vi "Keyence.Main.vi"(11 "idx":i32) -> ()   [LabVIEW 2016]
uses:
  Keyence.Data.ctl
  Keyence.Data.Status.ctl
  Keyence.Data.Status.State.ctl
  Keyence.Data.Sets.ctl
  LowLevel/Keyence.CodeDetails.ctl
  Keyence.Action.ctl
  tools/CitTemplate/citTemplate.errData.ctl
  tools/EventLog/EventLog.EventSource.ctl
  Global/ApplicationGlobal.vi
  LowLevel/Keyence.Global.vi
panel:
  out "Action":T1=enum."--- Keyence ---"
  out "Data":T2={"Status"={"State"=enum."Init", "Ref"=refnum, "Bank"=0, "Version"="", "Model"="", "EndTS"=timestamp(0 s since 1904-01-01), "ImgPath"=path "", "Tuned"=FALSE}, "Sets"={"IP"="192.168.2.1", "Timeout_ms"=5000, "Retries"=0, "ReconnectPeriod_s"=0, "ResetPeriod_s"=0, "ReadImg"=FALSE}, "Code"={"text"="", "status"=FALSE, "corners"=[], "level"=0, "class"="", "path"=path ""}}
  out "_loop":i32(ring)=4
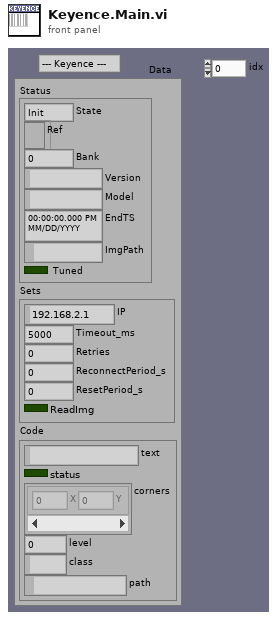
[diagram p1: front panel]
types:
  T1 = typedef "Keyence.Action.ctl" = enum32{"idle", "constructor", "destructor", "--- Keyence ---", "Init", "Scan", "Tune"}
  T2 = typedef "Keyence.Data.ctl" = cluster{"Status":T3, "Sets":T5, "Code":T6}
  T3 = typedef "Keyence.Data.Status.ctl" = cluster{"State":T4, "Ref":refnum<k5>, "Bank":u8, "Version":string, "Model":string, "EndTS":timestamp, "ImgPath":path, "Tuned":bool}
  T4 = typedef "Keyence.Data.Status.State.ctl" = enum16{"First", "Init", "Reset", "Idle", "Scan", "Tune"}
  T5 = typedef "Keyence.Data.Sets.ctl" = cluster{"IP":string, "Timeout_ms":i32, "Retries":i32, "ReconnectPeriod_s":i32, "ResetPeriod_s":i32, "ReadImg":bool}
  T6 = typedef "Keyence.CodeDetails.ctl" = cluster{"text":string, "status":bool, "corners":cluster{"X":i32, "Y":i32}[], "level":u8, "class":string, "path":path}
  T7 = typedef "EventLog.EventSource.ctl" = enum16{"All", "Gui", "Ref", "File", "Arch", "Seq", "CPX", "DB", "Laser", "Scan.P", "Scan.O"}
  T8 = typedef "citTemplate.errData.ctl" = cluster{"ts":timestamp, "src":T7, "instance":i32, "action":string, "error":errorcluster, "unconfirmed":bool}
  T9 = cluster{u8, "imgpath":path, "Retries (-1: Default)":i32, "get img":bool}
  T10 = typedef "citTemplate.notifierHandle.ctl" = refnum<notifier>
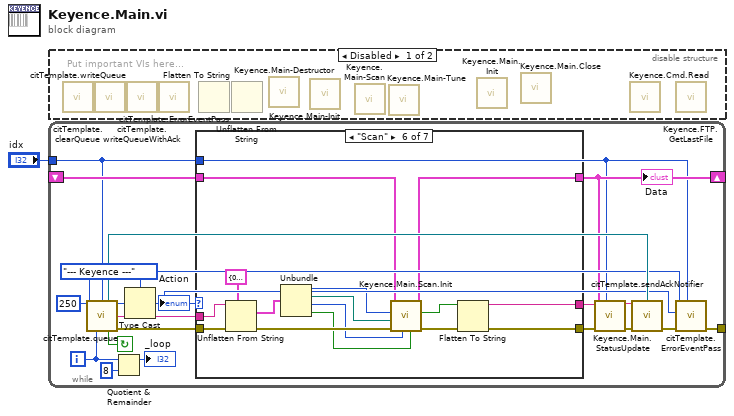
[diagram p0: block diagram]
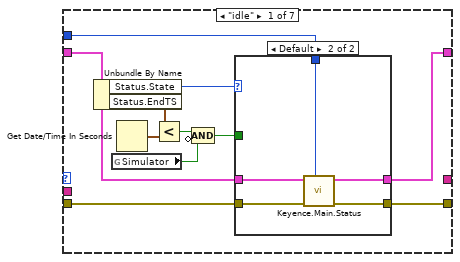
[diagram p3: hidden frame]
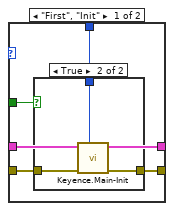
[diagram p4: hidden frame]
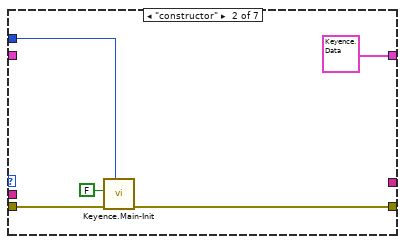
[diagram p6: hidden frame]
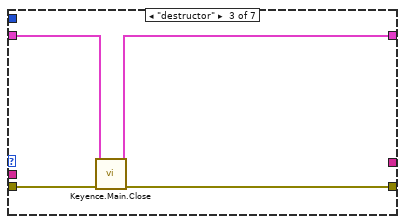
[diagram p7: hidden frame]
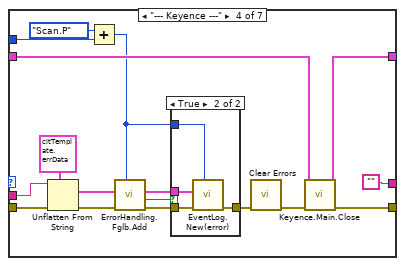
[diagram p8: hidden frame]
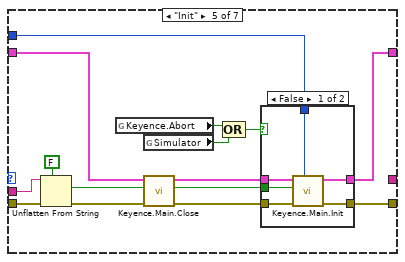
[diagram p10: hidden frame]
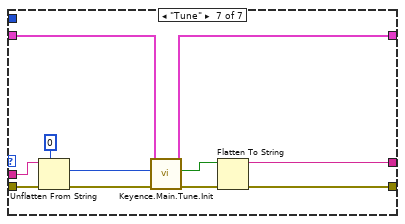
[diagram p12: hidden frame]
diagram:
  n1 = while {
    tunnel: [w10] -> _
    shift-right: [w3] -> _
    shift-left: _ -> [w7]
    tunnel: "idx" -> [w2]
    i -> [w6]
    stop <- w17 continue-if-true
    w5 = Keyence.Action."--- Keyence ---" ("Action")
    n2 = call "citTemplate.queue.vi"("ms timeout (250 ms)"=250, "instance (0)"=w2, "event enum"=w5, "iteration (-1)"=w6) -> ("notifierHandle out"=w16:T10, "event out"=w19:u32, "(flatten) data out"=w18:string, "continue"=w17:bool, "error out"=w8:errorcluster)  [unwired: 1 in, 6 out]
    n3 = Quotient & Remainder(x=w6, y=8) -> (x-y*floor(x/y)=→"_loop":i32)  [unwired: 1 out]
    n4 = Type Cast(type=w5, x=w19) -> (*(type *) &x=w11:T1)
    "Action" <- w11
    n5 = case shown="\"Scan\"" w11 {
      tunnel: w18 -> [_ _ _ w68 w78 w110 w121]
      tunnel: [_ _ _ "" _ w103 w114] -> w15
      tunnel: [w29 w48 w52 w60 w88 w105 w116] -> w14
      tunnel: [w26 T2 {"Status"={"State"=enum."First", "Ref"=refnum, "Bank"=0, "Version"="", "Model"="", "EndTS"=timestamp(0 s since 1904-01-01), "ImgPath"=path "", "Tuned"=FALSE}, "Sets"={"IP"="", "Timeout_ms"=0, "Retries"=0, "ReconnectPeriod_s"=0, "ResetPeriod_s"=0, "ReadImg"=FALSE}, "Code"={"text"="", "status"=FALSE, "corners"=[], "level"=0, "class"="", "path"=path ""}} ("Data") w50 w58 w85 w107 w118] -> w3
      tunnel: w8 -> [w30 w49 w53 w67 w79 w111 w122]
      tunnel: w7 -> [w27 _ w51 w59 w80 w108 w119]
      tunnel: w2 -> [w20 w46 _ w55 w81 _ _]
      frame "idle" {
        n6 = Unbundle By Name(w27) -> ("Status.State"=w28:T4, "Status.EndTS"=w25:timestamp)
        n7 = global read "ApplicationGlobal.vi" "Simulator"() -> (w21:bool)
        n8 = Get Date/Time In Seconds() -> (seconds since 1Jan1904=w24:timestamp)
        n9 = Less?(x=w25, y=w24) -> (x < y?=w23:bool)
        n10 = Compound Arithmetic op=AND(w23, invert w21) -> (w22:bool)
        n11 = case shown="Default" w28 {
          tunnel: w30 -> [w35 w44]
          tunnel: [w34 w41] -> w29
          tunnel: [w33 w43] -> w26
          tunnel: w27 -> [w33 w42]
          tunnel: w22 -> [w32 _]
          tunnel: w20 -> [w31 w40]
          frame "First", "Init" {
            n12 = case shown="True" w32 {
              tunnel: w35 -> [w36 w39]
              tunnel: [w36 w38] -> w34
              tunnel: w31 -> [_ w37]
              frame False {
              }
              frame True {
                n13 = call "Keyence.Main-Init.vi"("Idx"=w37, "error in"=w39) -> ("error out"=w38:errorcluster)  [unwired: 9 in]
              }
            }
          }
          frame Default {
            n14 = call "Keyence.Main.Status.vi"("Idx"=w40, "error in"=w44, "Data in"=w42) -> ("error out"=w41:errorcluster, "Data out"=w43:T2)  [unwired: 7 in]
          }
        }
      }
      frame "constructor" {
        n15 = call "Keyence.Main-Init.vi"("Idx"=w46, "error in"=w49, "restart (T)"=FALSE) -> ("error out"=w48:errorcluster)  [unwired: 8 in]
      }
      frame "destructor" {
        n16 = call "Keyence.Main.Close.vi"("error in"=w53, "Data in"=w51) -> ("error out"=w52:errorcluster, "Data out"=w50:T2)  [unwired: 8 in]
      }
      frame "--- Keyence ---" {
        n17 = Unflatten From String(type=T8 {"ts"=timestamp(0 s since 1904-01-01), "src"=enum."All", "instance"=0, "action"="", "error"={"status"=FALSE, "code"=0, "source"=""}, "unconfirmed"=FALSE} ("ErrData"), binary string=w68, error in (no error)=w67) -> (value=w63:T8, error out=w62:errorcluster)  [unwired: 3 out]
        n18 = Add(x=EventLog.EventSource."Scan.P" ("Event source"), y=w55) -> (x+y=w54:i32)
        n19 = call "ErrorHandling.Fglb.Add.vi"("Event source"=w54, "error in (no error)"=w62, "Error in"=w63) -> ("error out"=w65:errorcluster, "changed?"=w57:bool)  [unwired: 7 in]
        n20 = case shown="True" w57 {
          tunnel: w65 -> [w70 w74]
          tunnel: [w70 w73] -> w64
          tunnel: w54 -> [_ w72]
          tunnel: w63 -> [_ w71]
          frame False {
          }
          frame True {
            n21 = call "EventLog.New(error).vi"("Source (All)"=w72, "error in"=w74, "ErrData"=w71) -> ("error out"=w73:errorcluster)  [unwired: 8 in]
          }
        }
        n22 = call <vilib>:"Clear Errors.vi"("error in (no error)"=w64) -> ("error out"=w61:errorcluster)  [unwired: 5 in, 1 out]
        n23 = call "Keyence.Main.Close.vi"("error in"=w61, "Data in"=w59) -> ("error out"=w60:errorcluster, "Data out"=w58:T2)  [unwired: 8 in]
      }
      frame "Init" {
        n24 = Unflatten From String(type=FALSE, binary string=w78, error in (no error)=w79) -> (value=w75:bool, error out=w77:errorcluster)  [unwired: 2 in, 1 out]
        n25 = global read "Keyence.Global.vi" "Keyence.Abort"() -> (w84:bool)
        n26 = global read "ApplicationGlobal.vi" "Simulator"() -> (w82:bool)
        n27 = call "Keyence.Main.Close.vi"("error in"=w77, "Data in"=w80) -> ("error out"=w87:errorcluster, "Data out"=w86:T2)  [unwired: 8 in]
        n28 = Compound Arithmetic op=OR(w84, w82) -> (w83:bool)
        n29 = case shown="False" w83 {
          tunnel: [w94 w95] -> w88
          tunnel: w87 -> [w93 w95]
          tunnel: w86 -> [w92 w96]
          tunnel: [w91 w96] -> w85
          tunnel: w81 -> [w90 _]
          tunnel: w75 -> [w89 _]
          frame False {
            n30 = call "Keyence.Main.Init.vi"("Idx"=w90, "error in"=w93, "restart"=w89, "Data in"=w92) -> ("error out"=w94:errorcluster, "Data out"=w91:T2)  [unwired: 6 in]
          }
          frame True {
          }
        }
      }
      frame "Scan" {
        n31 = Unflatten From String(type=T9 {0, "imgpath"=path "", "Retries (-1: Default)"=0, "get img"=FALSE} ("output cluster"), binary string=w110, error in (no error)=w111) -> (value=w98:T9, error out=w109:errorcluster)  [unwired: 2 in, 1 out]
        n32 = Unbundle(w98) -> (w102:u8, "imgpath"=w101:path, "Retries (-1: Default)"=w100:i32, "get img"=w97:bool)
        n33 = call "Keyence.Main.Scan.Init.vi"("get image"=w97, "Retries (-1: Default)"=w100, "error in"=w109, "ImgPath"=w101, "Bank"=w102, "Data in"=w108) -> ("error out"=w106:errorcluster, "started"=w104:bool, "Data out"=w107:T2)  [unwired: 3 in]
        n34 = Flatten To String(anything=w104, error in (no error)=w106) -> (data string=w103:string, error out=w105:errorcluster)  [unwired: 2 in, 1 out]
      }
      frame "Tune" {
        n35 = Unflatten From String(type=u8 0, binary string=w121, error in (no error)=w122) -> (value=w112:u8, error out=w120:errorcluster)  [unwired: 2 in, 1 out]
        n36 = call "Keyence.Main.Tune.Init.vi"("error in"=w120, "Bank"=w112, "Data in"=w119) -> ("error out"=w117:errorcluster, "started"=w115:bool, "Data out"=w118:T2)  [unwired: 6 in]
        n37 = Flatten To String(anything=w115, error in (no error)=w117) -> (data string=w114:string, error out=w116:errorcluster)  [unwired: 2 in, 1 out]
      }
    }
    "Data" <- w3
    n38 = call "Keyence.Main.StatusUpdate.vi"("Idx"=w2, "error in"=w14, "Data in"=w3) -> ("error out"=w4:errorcluster)  [unwired: 8 in]
    n39 = call "citTemplate.sendAckNotifier.vi"("notification data"=w15, "notifierHandle in"=w16, "error in"=w4) -> ()  [unwired: 13 out]
    n40 = call "citTemplate.ErrorEventPass.vi"("instance"=w2, "error in"=w4, "action of error"=w11, "event in"=w5) -> ("error out"=w10:errorcluster)  [unwired: 1 in, 6 out]
  }
  n41 = disable-structure shown="Disabled" {
    frame Disabled {
      # "Put important VIs here..."
      n42 = call "citTemplate.clearQueue.vi"() -> ()  [unwired: 14 in, 2 out]
      n43 = call "citTemplate.writeQueue.vi"() -> ()  [unwired: 15 in, 1 out]
      n44 = call "citTemplate.writeQueueWithAck.vi"() -> ()  [unwired: 13 in, 3 out]
      n45 = call "citTemplate.ErrorEventPass.vi"() -> ()  [unwired: 11 in, 1 out]
      n46 = Flatten To String() -> ()  [unwired: 4 in, 3 out]
      n47 = Unflatten From String() -> ()  [unwired: 5 in, 3 out]
      n48 = call "Keyence.Main-Destructor.vi"() -> ()  [unwired: 11 in, 1 out]
      n49 = call "Keyence.Main-Init.vi"() -> ()  [unwired: 11 in, 1 out]
      n50 = call "Keyence.Main-Scan.vi"() -> ()  [unwired: 9 in, 3 out]
      n51 = call "Keyence.Main-Tune.vi"() -> ()  [unwired: 8 in, 4 out]
      n52 = call "Keyence.Main.Init.vi"() -> ()  [unwired: 10 in, 2 out]
      n53 = call "Keyence.Main.Close.vi"() -> ()  [unwired: 10 in, 2 out]
      n54 = call "Keyence.Cmd.Read.vi"() -> ()  [unwired: 8 in, 4 out]
      n55 = call "Keyence.FTP.GetLastFile.vi"() -> ()  [unwired: 10 in, 2 out]
    }
    frame Enabled {
    }
  }
